vi "getLaserPower.vi"(1 "laser":T1) -> (0 "laserPower (mW)":dbl)   [LabVIEW 2015]
uses:
  <vilib>/regexp/Match Regular Expression.xnode
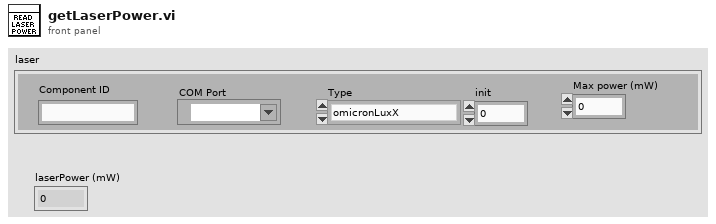
[diagram p1: front panel]
types:
  T1 = cluster{"Component ID":string, "COM Port":refnum<visa-resource-name>, "Type ":enum16{"omicronLuxX", "coherentObis"}, "init":i16, "Max power (mW)":dbl}
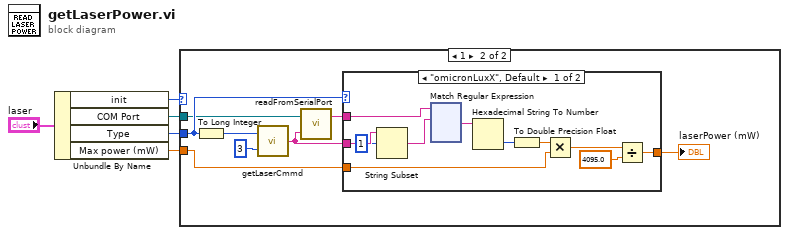
[diagram p0: block diagram]
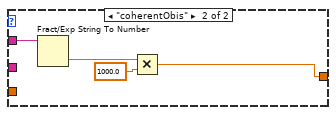
[diagram p3: hidden frame]
diagram:
  n1 = Unbundle By Name("laser") -> ("init"=w3:i16, "COM Port"=w4:refnum<visa-resource-name>, "Type"=w2:enum16{"omicronLuxX", "coherentObis"}, "Max power (mW)"=w1:dbl)
  n2 = case shown="1" w3 {
    tunnel: w4 -> [_ w10]
    tunnel: w2 -> [_ w11]
    tunnel: w1 -> [_ w8]
    frame 0, Default {
    }
    frame 1 {
      n3 = To Long Integer(number=w11) -> (32bit integer=w12:i32)
      n4 = call "getLaserCmmd.vi"("Cmmd index"=3, "Laser type"=w12) -> ("Laser command"=w6:string)
      n5 = call "readFromSerialPort.vi"("Cmmd"=w6, "input COM Port"=w10) -> ("read buffer"=w9:string)  [unwired: 1 out]
      n6 = case shown="\"omicronLuxX\", Default" w11 {
        tunnel: w9 -> [w14 w140]
        tunnel: w8 -> [w20 _]
        tunnel: [w18 w139] -> w7
        tunnel: w6 -> [w17 _]
        frame "omicronLuxX", Default {
          n7 = String Subset(string=w17, offset (0)=1) -> (substring=w15:string)  [unwired: 1 in]
          n8 = xnode "Match Regular Expression"("input string"=w14, "regular expression"=w15) -> ("after match"=w19:string)  [unwired: 4 in, 4 out]
          n9 = Hexadecimal String To Number(string=w19) -> (number=w24:u32)  [unwired: 2 in, 1 out]
          n10 = To Double Precision Float(number=w24) -> (double precision float=w23:dbl)
          n11 = Multiply(x=w23, y=w20) -> (x*y=w21:dbl)
          n12 = Divide(x=w21, y=4095.0) -> (x/y=w18:dbl)
        }
        frame "coherentObis" {
          n13 = Fract/Exp String To Number(string=w140) -> (number=w141:dbl)  [unwired: 3 in, 1 out]
          n14 = Multiply(x=w141, y=1000.0) -> (x*y=w139:dbl)
        }
      }
      "laserPower (mW)" <- w7
    }
  }
